vi "End Group.vi"(8 "error in (no error)":errorcluster {"code" format="Error %.0f"}, 10 "Group":string, 11 "VIDoc Printer - Confluence In":refnum<class "VIDoc Printer - Confluence.lvclass">) -> (0 "error out":errorcluster {"code" format="Error %.0f"}, 3 "VIDoc Printer - Confluence Out":refnum<class "VIDoc Printer - Confluence.lvclass">)   [LabVIEW 2023, in "VIDoc Printer - Confluence.lvlib" / "VIDoc Printer - Confluence.lvclass"]
uses:
  VIDoc Printer - Confluence.lvclass
  Printer/VIDoc Printer.lvclass
  VIDoc Printer - Confluence.lvclass/VIDoc Printer - Confluence.ctl
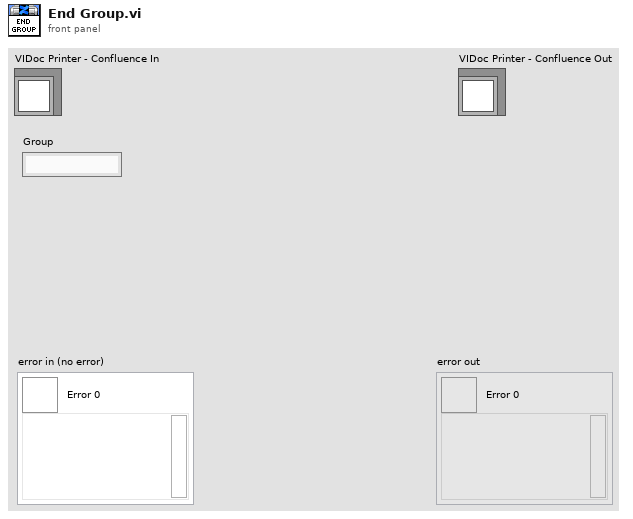
[diagram p1: front panel]
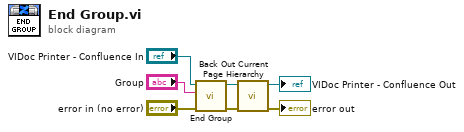
[diagram p0: block diagram]
diagram:
  n1 = call-parent "End Group.vi"("error in (no error)"="error in (no error)", "Group"="Group", "VIDoc Printer In"="VIDoc Printer - Confluence In") -> ("error out"=w3:errorcluster, "VIDoc Printer Out"=w4:refnum<class "VIDoc Printer - Confluence.lvclass">)  [unwired: 7 in]
  n2 = call "Back Out Current Page Hierarchy.vi"("error in (no error)"=w3, "VIDoc Printer - Confluence In"=w4) -> ("error out"=→"error out":errorcluster, "VIDoc Printer - Confluence Out"=→"VIDoc Printer - Confluence Out":refnum<class "VIDoc Printer - Confluence.lvclass">)  [unwired: 8 in]
